vi "Control.vi"(8 "Parallel Output":dbl, 9 "Process Variable":dbl, 10 "Setpoint":dbl, 11 "PI-Controller in":T1) -> (2 "Output":dbl, 3 "PID out":T1)   [LabVIEW 2015, in "PID.lvlib"]
uses:
  PID.lvlib
  PID.ctl
  Anti-Windup Method.ctl
  Gains.ctl
  Output Range.ctl
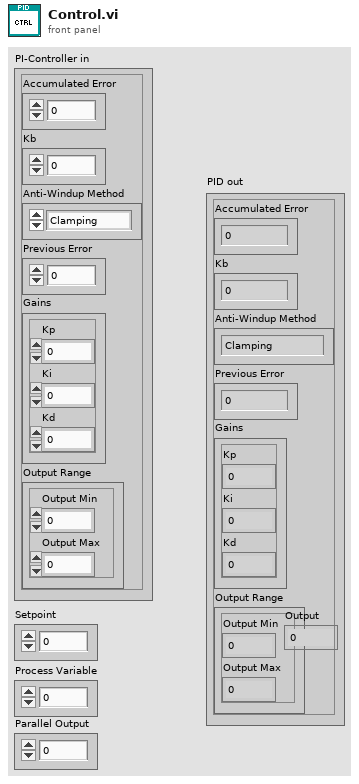
[diagram p1: front panel]
types:
  T1 = typedef "PID.lvlib/PID.ctl" = cluster{"Accumulated Error":dbl, "Kb":dbl, "Anti-Windup Method":T2, "Previous Error":dbl, "Gains":T3, "Output Range":T4}
  T2 = typedef "PID.lvlib/Anti-Windup Method.ctl" = enum16{"Clamping", "Back-Calculation", "None"}
  T3 = typedef "PID.lvlib/Gains.ctl" = cluster{"Kp":dbl, "Ki":dbl, "Kd":dbl}
  T4 = typedef "PID.lvlib/Output Range.ctl" = cluster{"Output Min":dbl, "Output Max":dbl}
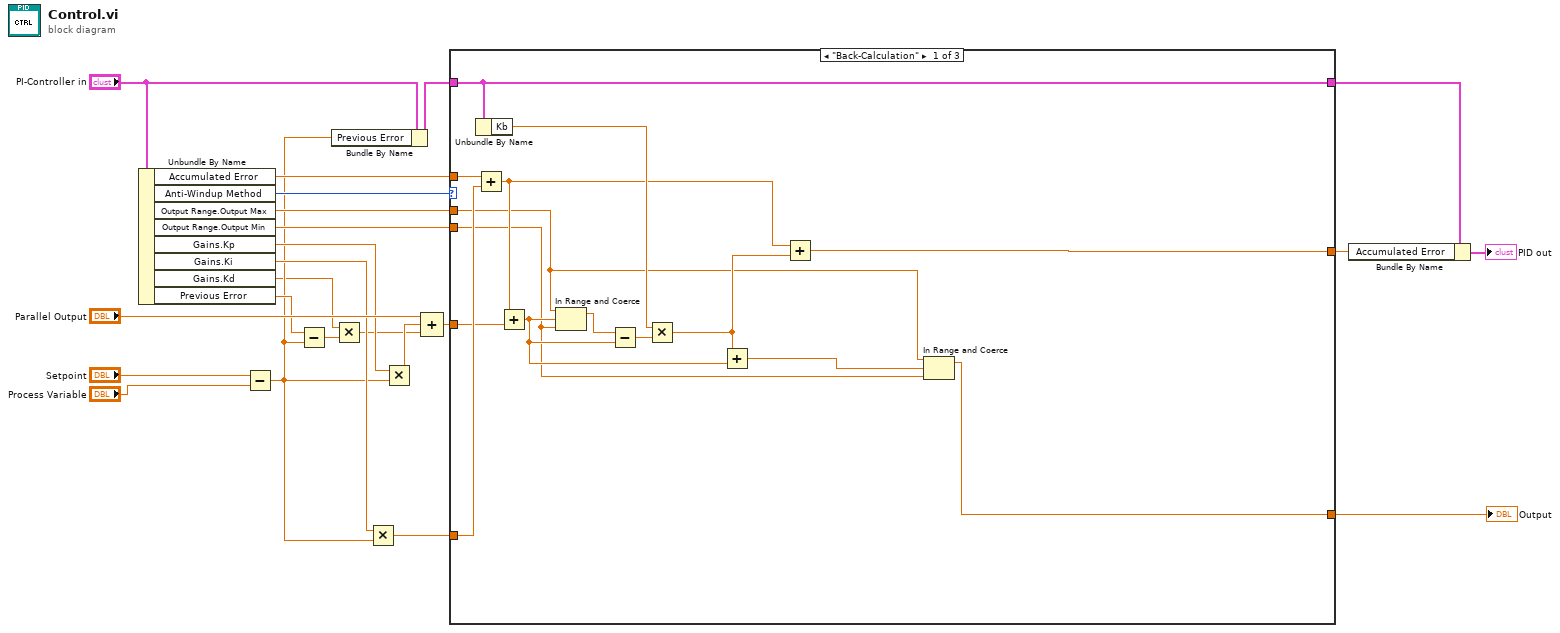
[diagram p0: block diagram]
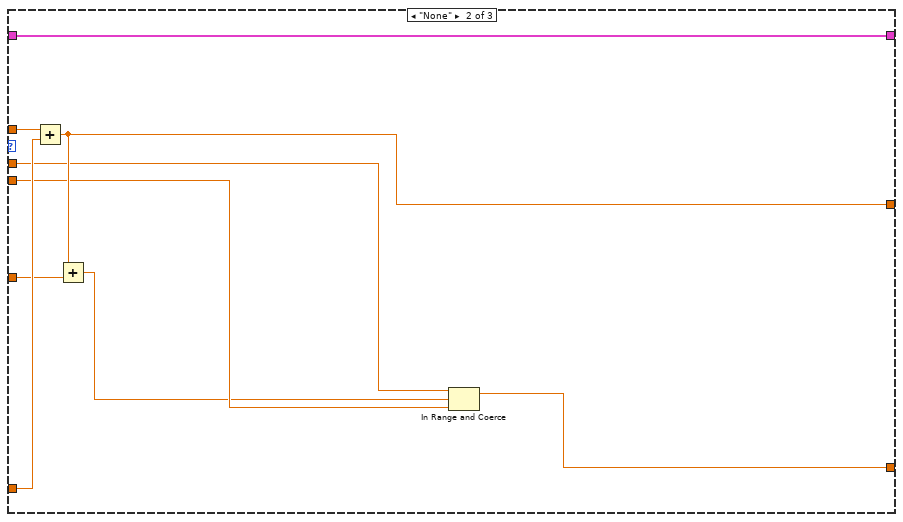
[diagram p2: hidden frame]
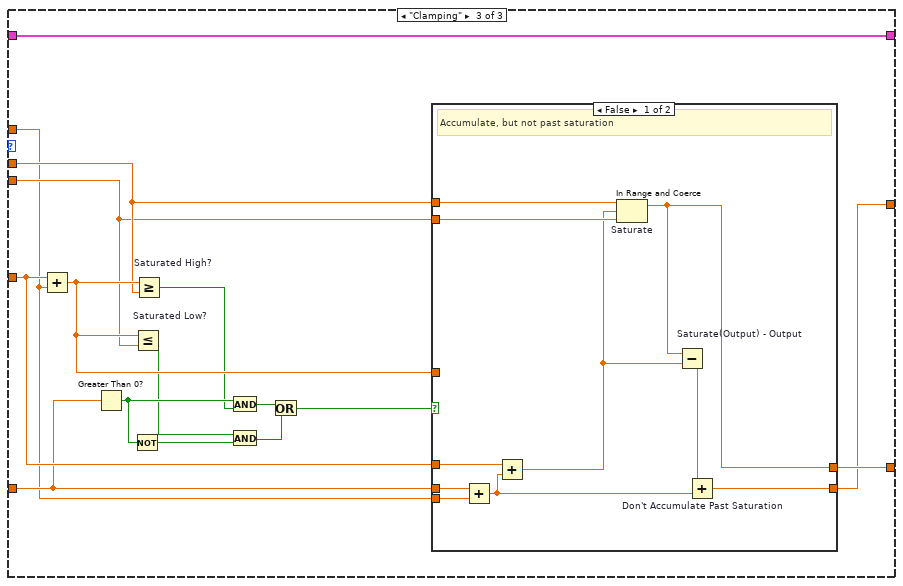
[diagram p3: hidden frame]
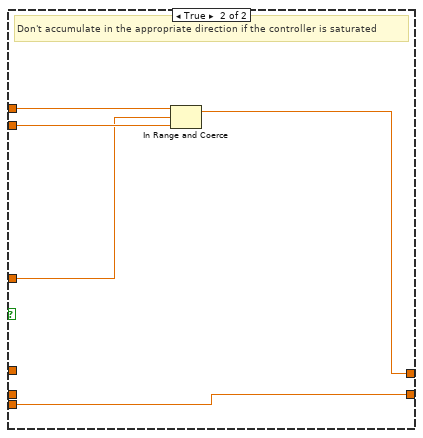
[diagram p4: hidden frame]
diagram:
  n1 = Unbundle By Name("PI-Controller in") -> ("Accumulated Error"=w11:dbl, "Anti-Windup Method"=w12:T2, "Output Range.Output Max"=w20:dbl, "Output Range.Output Min"=w19:dbl, "Gains.Kp"=w15:dbl, "Gains.Ki"=w14:dbl, "Gains.Kd"=w3:dbl, "Previous Error"=w5:dbl)
  n2 = Subtract(x="Setpoint", y="Process Variable") -> (x-y=w4:dbl)
  n3 = Subtract(x=w5, y=w4) -> (x-y=w2:dbl)
  n4 = Bundle By Name(cluster="PI-Controller in", "Previous Error"=w4) -> (w6:T1)
  n5 = Multiply(x=w3, y=w2) -> (x*y=w1:dbl)
  n6 = Multiply(x=w14, y=w4) -> (x*y=w21:dbl)
  n7 = Multiply(x=w15, y=w4) -> (x*y=w22:dbl)
  n8 = Compound Arithmetic op=ADD("Parallel Output", w22, w1) -> (w23:dbl)
  n9 = case shown="\"Back-Calculation\"" w12 {
    tunnel: w23 -> [w36 w45 w62]
    tunnel: w21 -> [w37 w46 w60]
    tunnel: w20 -> [w27 w42 w53]
    tunnel: w19 -> [w26 w41 w52]
    tunnel: [w24 w39 w51] -> w13
    tunnel: w11 -> [w38 w47 w49]
    tunnel: [w28 w44 w50] -> w9
    tunnel: w6 -> [w31 w43 w48]
    tunnel: [w31 w43 w48] -> w8
    frame "Back-Calculation" {
      n10 = Unbundle By Name(w31) -> ("Kb"=w33:dbl)
      n11 = Add(x=w38, y=w37) -> (x+y=w29:dbl)
      n12 = Add(x=w29, y=w36) -> (x+y=w32:dbl)
      n13 = In Range and Coerce(upper limit=w27, x=w32, lower limit=w26) -> (coerced(x)=w35:dbl)  [unwired: 1 out]
      n14 = Subtract(x=w35, y=w32) -> (x-y=w34:dbl)
      n15 = Multiply(x=w33, y=w34) -> (x*y=w30:dbl)
      n16 = Add(x=w30, y=w32) -> (x+y=w25:dbl)
      n17 = Add(x=w29, y=w30) -> (x+y=w28:dbl)
      n18 = In Range and Coerce(upper limit=w27, x=w25, lower limit=w26) -> (coerced(x)=w24:dbl)  [unwired: 1 out]
    }
    frame "None" {
      n19 = Add(x=w47, y=w46) -> (x+y=w44:dbl)
      n20 = Add(x=w44, y=w45) -> (x+y=w40:dbl)
      n21 = In Range and Coerce ("Saturate")(upper limit=w42, x=w40, lower limit=w41) -> (coerced(x)=w39:dbl)  [unwired: 1 out]
    }
    frame "Clamping" {
      n22 = Add(x=w62, y=w49) -> (x+y=w63:dbl)
      n23 = Greater Than 0?(x=w60) -> (x > 0?=w57:bool)
      n24 = Not(x=w57) -> (.not. x?=w56:bool)
      n25 = Less Or Equal? "Saturated Low?"(x=w63, y=w52) -> (x <= y?=w55:bool)
      n26 = Greater Or Equal? "Saturated High?"(x=w63, y=w53) -> (x >= y?=w54:bool)
      n27 = And(x=w57, y=w54) -> (x .and. y?=w58:bool)
      n28 = And(x=w55, y=w56) -> (x .and. y?=w59:bool)
      n29 = Or(x=w58, y=w59) -> (x .or. y?=w61:bool)
      n30 = case shown="False" w61 {
        tunnel: w60 -> [w73 _]
        tunnel: w49 -> [w72 w78]
        tunnel: w62 -> [w71 _]
        tunnel: w53 -> [w70 w77]
        tunnel: w52 -> [w69 w76]
        tunnel: [w67 w78] -> w50
        tunnel: [w64 w74] -> w51
        tunnel: w63 -> [_ w75]
        frame False {
          # "Accumulate, but not past saturation"
          n31 = Add(x=w73, y=w72) -> (x+y=w65:dbl)
          n32 = Add(x=w71, y=w65) -> (x+y=w66:dbl)
          n33 = In Range and Coerce "Saturate"(upper limit=w70, x=w66, lower limit=w69) -> (coerced(x)=w64:dbl)  [unwired: 1 out]
          n34 = Subtract "Saturate(Output) - Output"(x=w64, y=w66) -> (x-y=w68:dbl)
          n35 = Add "Don't Accumulate Past Saturation"(x=w68, y=w65) -> (x+y=w67:dbl)
        }
        frame True {
          # "Don't accumulate in the appropriate direction if the controller is saturated"
          n36 = In Range and Coerce(upper limit=w77, x=w75, lower limit=w76) -> (coerced(x)=w74:dbl)  [unwired: 1 out]
        }
      }
    }
  }
  "Output" <- w13
  n37 = Bundle By Name(cluster=w8, "Accumulated Error"=w9) -> (→"PID out":T1)
